vi "Ramp Timer.vi"(0 "Previous Ramp Time":u32) -> (1 "New Start Time":u32, 2 "Current Ramp Time":u64)   [LabVIEW 2009]
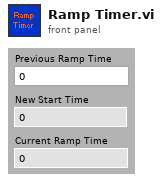
[diagram p1: front panel]
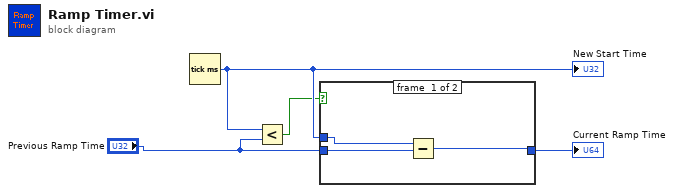
[diagram p0: block diagram]
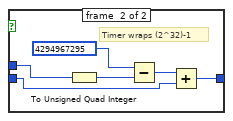
[diagram p2: hidden frame]
diagram:
  n1 = Tick Count (ms)() -> (millisecond timer value=w4:u32)
  "New Start Time" <- w4
  n2 = Less?(x=w4, y="Previous Ramp Time") -> (x < y?=w1:bool)
  n3 = case shown="False" w1 {
    tunnel: w4 -> [w6 w13]
    tunnel: "Previous Ramp Time" -> [w5 w11]
    tunnel: [w7 w10] -> w3
    frame #0 {
      n4 = Subtract(x=w6, y=w5) -> (x-y=w7:u32)
    }
    frame #1 {
      # "Timer wraps (2^32)-1"
      n5 = To Unsigned Quad Integer(1:w13) -> (0:w8:u64)
      n6 = Subtract(x=u64 4294967295, y=w8) -> (x-y=w12:u64)
      n7 = Add(x=w12, y=w11) -> (x+y=w10:u64)
    }
  }
  "Current Ramp Time" <- w3
